vi "Write Element of OVP Limit.vi"(8 "error in (no error)":errorcluster, 9 "limit (0.0 Volts)":dbl[unit] format="%^.2e", 10 "index":i32, 11 "CS++DCPwrChannelData in":refnum<class "CS++DCPwrChannelData.lvclass">) -> (0 "error out":errorcluster, 3 "CS++DCPwrChannelData out":refnum<class "CS++DCPwrChannelData.lvclass">)   [LabVIEW 2016, in "CS++DCPwrGui.lvlib" / "CS++DCPwrChannelData.lvclass"]
uses:
  CS++DCPwrChannelData.lvclass
  CS++DCPwrChannelData.lvclass/CS++DCPwrChannelData.ctl
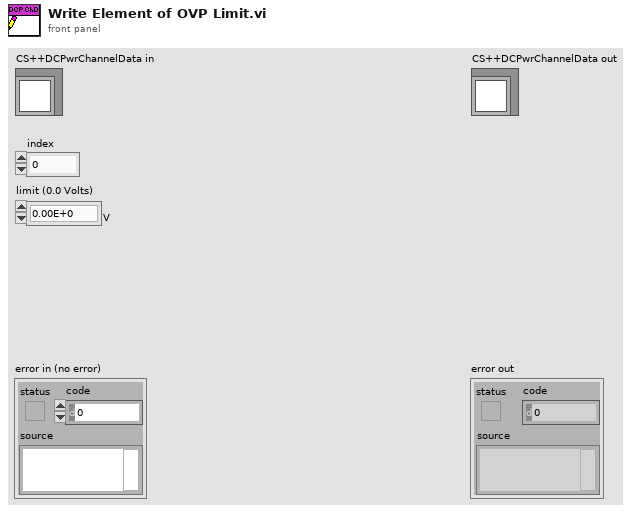
[diagram p1: front panel]
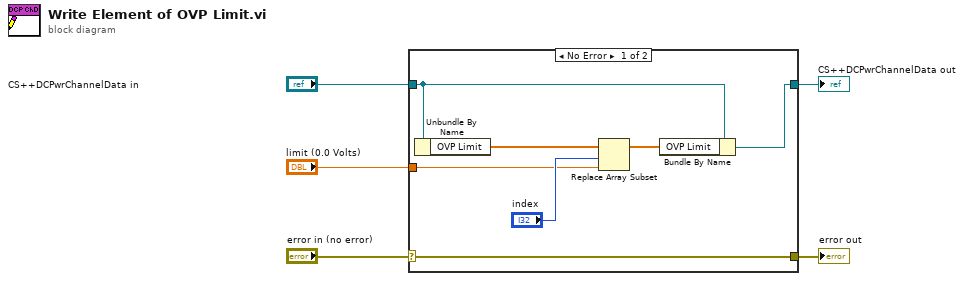
[diagram p0: block diagram]
diagram:
  n1 = case shown="No Error" "error in (no error)" {
    selector: "error in (no error)" -> [w12 w13]
    tunnel: [w12 w13] -> w4
    tunnel: [w11 w14] -> w2
    tunnel: "CS++DCPwrChannelData in" -> [w10 w14]
    tunnel: "limit (0.0 Volts)" -> [w6 _]
    frame No Error {
      n2 = Unbundle By Name(w10) -> ("OVP Limit"=w9:dbl[unit][])
      n3 = Replace Array Subset(array=w9, new element=w6, index="index") -> (w8:dbl[unit][])
      n4 = Bundle By Name(cluster=w10, "OVP Limit"=w8) -> (w11:refnum<class "CS++DCPwrChannelData.lvclass">)
    }
    frame Error {
    }
  }
  "error out" <- w4
  "CS++DCPwrChannelData out" <- w2
